vi "dddd.vi"() -> ()   [LabVIEW 2010]
uses:
  <vilib>/NXT/Block Support/NXT_InputPort.ctl
  <vilib>/NXT/Block Support/NXT_OutputPort.ctl
  <vilib>/NXT/Subs/MotorOutput.ctl
  <vilib>/NXT/Dual Mode Library/Sensors/Sonar_cm.vi
  <vilib>/NXT/Dual Mode Library/Motors/MotorOn.vi
  <vilib>/NXT/Dual Mode Library/Waits/Wait_Rotation.vi
panel:
  in  "stop":bool
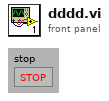
[diagram p1: front panel]
types:
  T1 = typedef "NXT_InputPort.ctl" = u8
  T2 = typedef "MotorOutput.ctl" = u8
  T3 = typedef "NXT_OutputPort.ctl" = u8
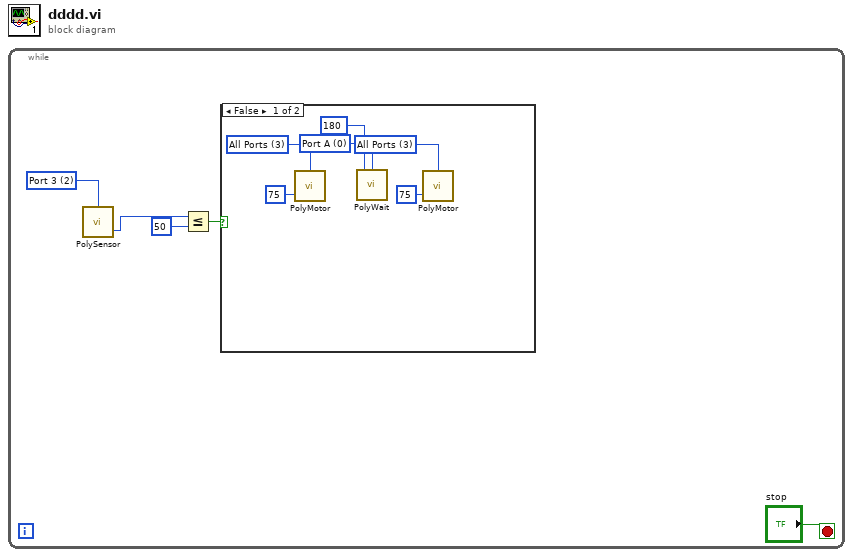
[diagram p0: block diagram]
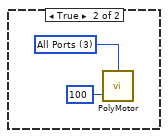
[diagram p2: hidden frame]
diagram:
  n1 = while {
    stop <- "stop" stop-if-true
    w5 = T1 2 items=["Port 1", "Port 2", "Port 3", "Port 4"] ("Port (Port 4)")
    n2 = call-poly <vilib>:"PolySensor.vi"("Port (Port 4)"=w5) -> ("Distance (cm)"=w4:i16)  [unwired: 2 in, 1 out]
    n3 = Less Or Equal?(x=w4, y=i16 50) -> (x <= y?=w2:bool)
    n4 = case shown="False" w2 {
      frame False {
        w9 = T2 3 items=["Port A", "Port B", "Port C", "All Ports"] ("Output Port (All Ports)")
        w10 = T3 0 items=["Port A", "Port B", "Port C"] ("Port (Port A)")
        w11 = T2 3 items=["Port A", "Port B", "Port C", "All Ports"] ("Output Port (All Ports)")
        n5 = call-poly <vilib>:"PolyMotor.vi"("Power (75)"=75, "Output Port (All Ports)"=w11) -> ()  [unwired: 2 in, 1 out]
        n6 = call-poly <vilib>:"PolyWait.vi"("Position Change (180)"=180, "Port (Port A)"=w10) -> ()  [unwired: 2 in, 1 out]
        n7 = call-poly <vilib>:"PolyMotor.vi"("Power (75)"=75, "Output Port (All Ports)"=w9) -> ()  [unwired: 2 in, 1 out]
      }
      frame True {
        w13 = T2 3 items=["Port A", "Port B", "Port C", "All Ports"] ("Output Port (All Ports)")
        n8 = call-poly <vilib>:"PolyMotor.vi"("Power (75)"=100, "Output Port (All Ports)"=w13) -> ()  [unwired: 2 in, 1 out]
      }
    }
  }
